vi "Sensor Interface - Fire Deposit.vi"(8 "error in (no error)":errorcluster, 10 "Deposit Received":bool, 11 "View Model":T1) -> (0 "error out":errorcluster, 3 "View Model":T1)   [LabVIEW 2017]
doc: "Generates User Event when Deposit received"
uses:
  View Model/Controls/View Model.ctl
  Error Handler/Controls/Error Model.ctl
  Error Handler/Controls/Error Data.ctl
  Error Handler/Controls/Error Type.ctl
  View Model/Controls/Shared Model.ctl
  Configuration/Controls/Config Model.ctl
  Configuration/Controls/Config CMD.ctl
  Configuration/Controls/Config Data.ctl
  ATM Controller/Controls/Controller Model.ctl
  ATM Controller/Controls/Controller Overhead.ctl
  ATM Controller/Controls/Controller States.ctl
  User Console View/Controls/User Console - Keypad.ctl
  User Console View/Controls/User Console - Transactions.ctl
  ATM Controller/Controls/Controller CMD.ctl
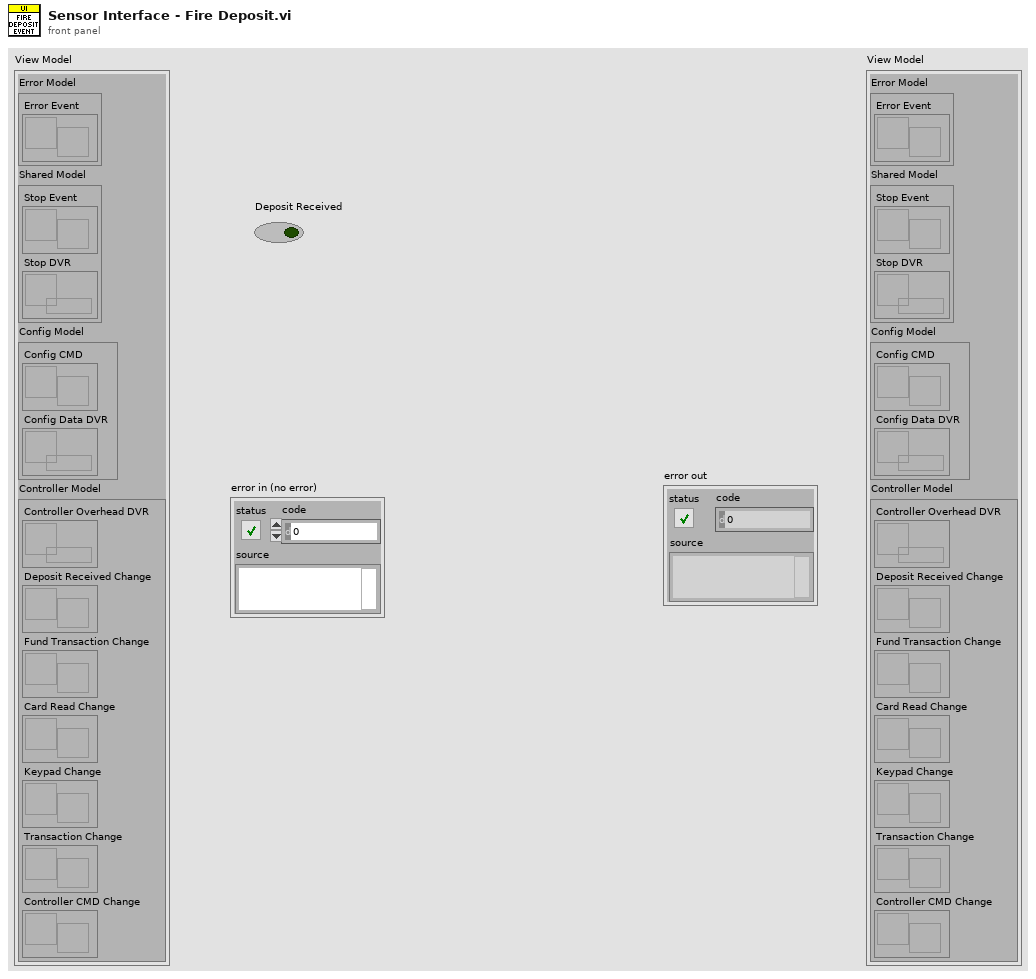
[diagram p1: front panel]
types:
  T1 = typedef "View Model.ctl" = cluster{"Error Model":T2, "Shared Model":T3, "Config Model":T4, "Controller Model":T5}
  T2 = typedef "Error Model.ctl" = cluster{"Error Event":refnum<user-event>}
  T3 = typedef "Shared Model.ctl" = cluster{"Stop Event":refnum<user-event>, "Stop DVR":refnum<data-value>}
  T4 = typedef "Config Model.ctl" = cluster{"Config CMD":refnum<user-event>, "Config Data DVR":refnum<data-value>}
  T5 = typedef "Controller Model.ctl" = cluster{"Controller Overhead DVR":refnum<data-value>, "Deposit Received Change":refnum<user-event>, "Fund Transaction Change":refnum<user-event>, "Card Read Change":refnum<user-event>, "Keypad Change":refnum<user-event>, "Transaction Change":refnum<user-event>, "Controller CMD Change":refnum<user-event>}
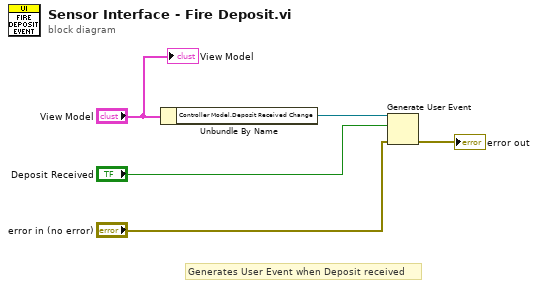
[diagram p0: block diagram]
diagram:
  # "Generates User Event when Deposit received"
  n1 = Unbundle By Name("View Model") -> ("Controller Model.Deposit Received Change"=w5:refnum<user-event>)
  n2 = Generate User Event(user event=w5, event data cluster="Deposit Received", error in="error in (no error)") -> (error out=→"error out":errorcluster)  [unwired: 1 in, 1 out]
  "View Model" <- "View Model"
